vi "TimeTag_LSW_AG_edits_May9.vi"() -> ()   [LabVIEW 2015]
doc: "This sample project is built upon the standard state machine template and shows how you could create an application that acquires, analyzes, and presents data. It includes functionality for presenting configuration dialogs, preserving settings between executions, loading and saving data, as well as exporting graph images and text files.\n\nIt is most appropriate for data that is acquired instantly as it does not allow for screen updates mid acquisition nor does it allow for continuous streaming to disk."
uses:
  <vilib>/ptbypt/NI_PtbyPt.lvlib
panel:
  out "real coin/sec X point average":dbl
  out "Real coin cps X point average":dbl(graph)
  in  "number of points to average real c/s":dbl=100.0
  out "Ch4 100sec avg":dbl
  out "Ch2 100 sec avg":dbl
  out "real coin cps 100 pt\n avg":dbl
  out "all coin cps":dbl
  out "real coin cps":dbl
  out "random coin cps":dbl
  out "Real coin cps":dbl(graph)
  out "total coin/sec - total random coin/sec":dbl
  out "total random coincidences/sec":dbl
  out "Total Coin per sec":dbl
  out "Ch2/4 coin/sec":dbl(graph)
  out "Ch2/4 Total Coincidences":dbl
  out "Channel 2 CPS":dbl(graph)
  out "Channel 4 CPS":dbl(graph)
  out "Total Ch2 CPS":dbl
  out "Total Ch4 CPS":dbl
  in  "Averaging":dbl=10.0
  in  "Runs":dbl=100.0
  in  "Pulse TTL 2":bool
  in  "Pulse TTL 1":bool
  in  "Toggle\nTTL 2":bool
  in  "Toggle\nTTL 1":bool
  out "Total Starts":dbl
  in  "Record data":bool
  out "Initial time":dbl
  out "Elapsed time (s)":dbl
  out "FPGA_Run Status":dbl
  out "USB_Open Status":dbl
  out "Channel 4 Total\nCounts":dbl
  out "Channel 3 Total\nCounts":dbl
  out "Channel 2 Total\nCounts":dbl
  out "Channel 1 Total\nCounts":dbl
  in  "File Name":string="C:\\FPGA\\test.txt"
  out "?":dbl
  out "?":dbl
  out "?":dbl
  out "?":dbl
  out "stats":i64[](array[numeric])
  in  "Stop":bool
  out "Channel 4 CPS":dbl(knob) scale=0.0..2000000.0
  out "Channel 3 CPS":dbl(knob) scale=0.0..600.0
  out "Channel 2 CPS":dbl(knob) scale=0.0..700.0
  out "Channel 1 CPS":dbl(knob) scale=0.0..600.0
  # "Starts"
  # "Channel 1"
  # "Channel 2"
  # "Channel 3"
  # "Channel 4"
  # "Coincidence Channels 1 & 2"
  # "Coincidence Channels 1 & 3"
  # "Coincidence Channels 1 & 4"
  # "Coincidence Channels 2 & 3"
  # "Coincidence Channels 2 & 4"
  # "Coincidence Channels 3 & 4"
  # "Coincidence Channels 1 & 2 & 3"
  # "Coincidence Channels 1 & 2 & 4"
  # "Coincidence Channels 1 & 3 & 4"
  # "Coincidence Channels 2 & 3 & 4"
  # "C:\\FPGA_Lauren"
  # "Coincidence Channels 1 & 2 & 3 & 4"
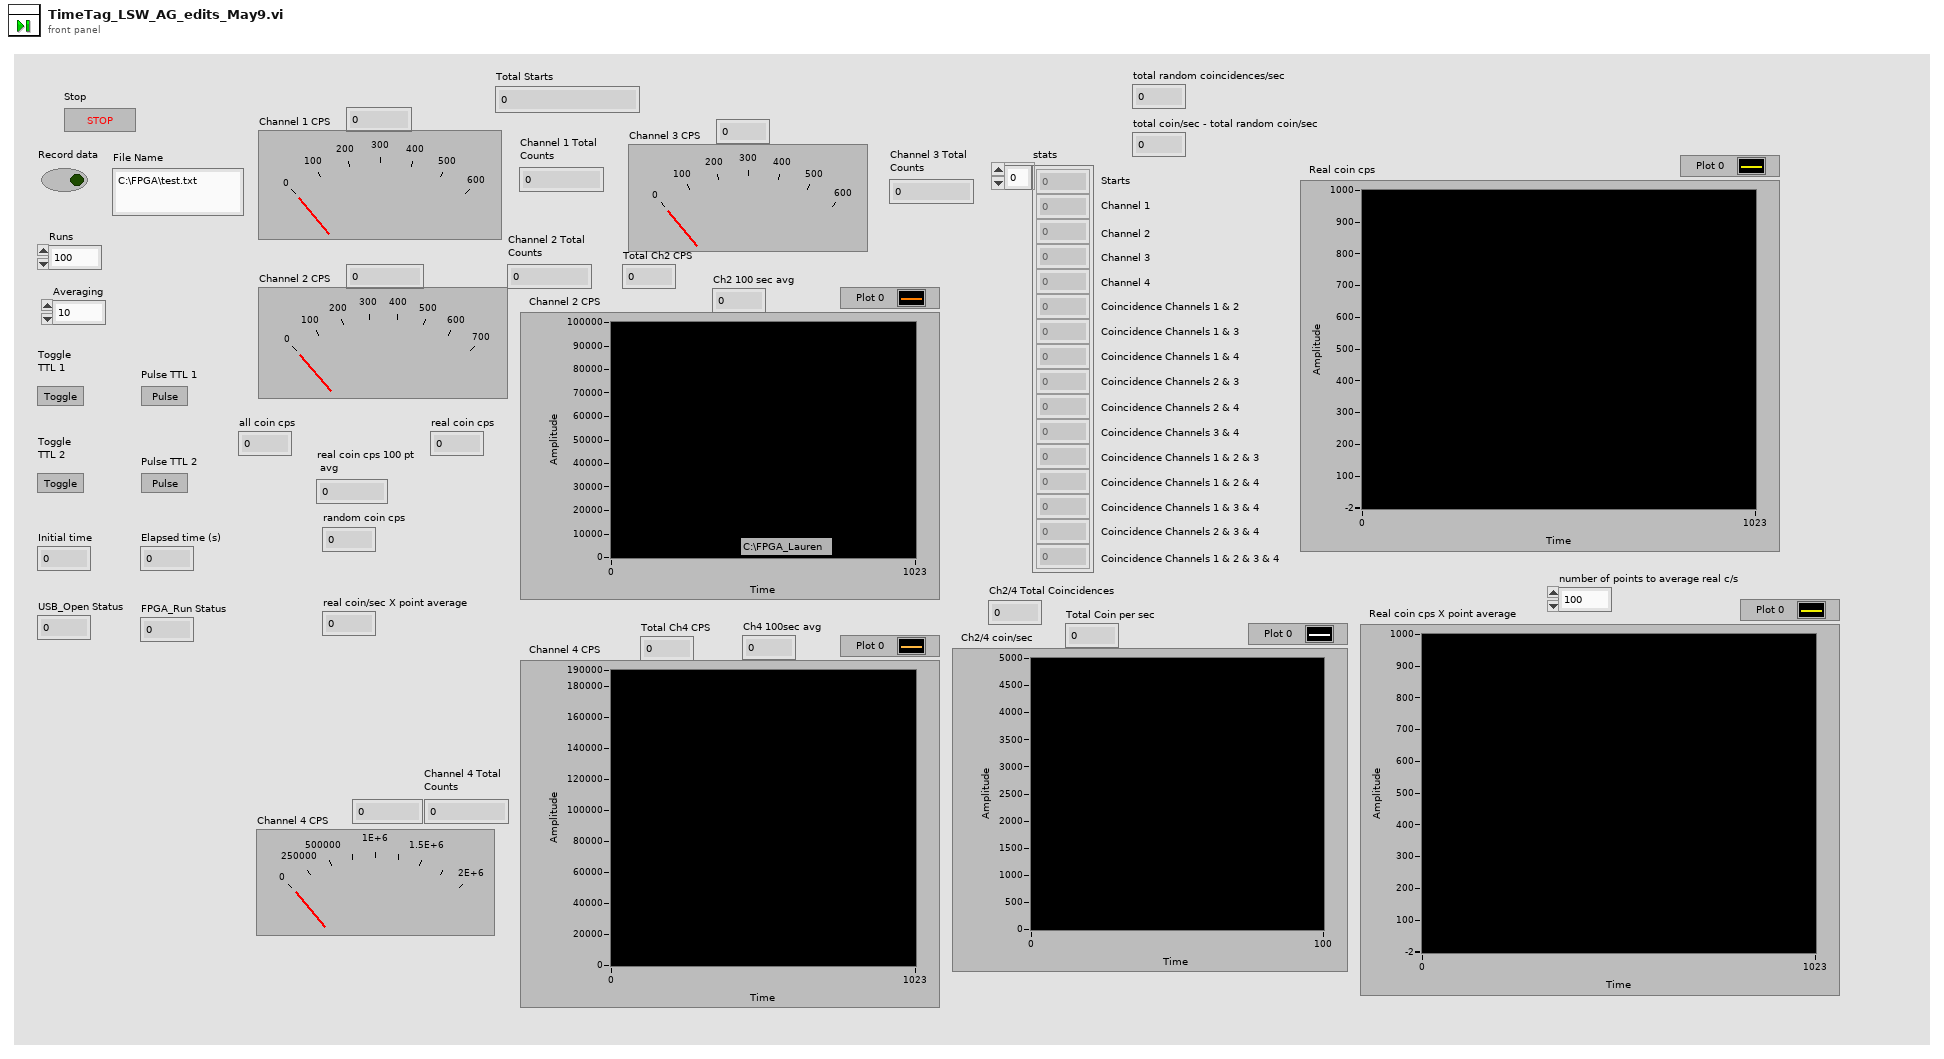
[diagram p1: front panel]
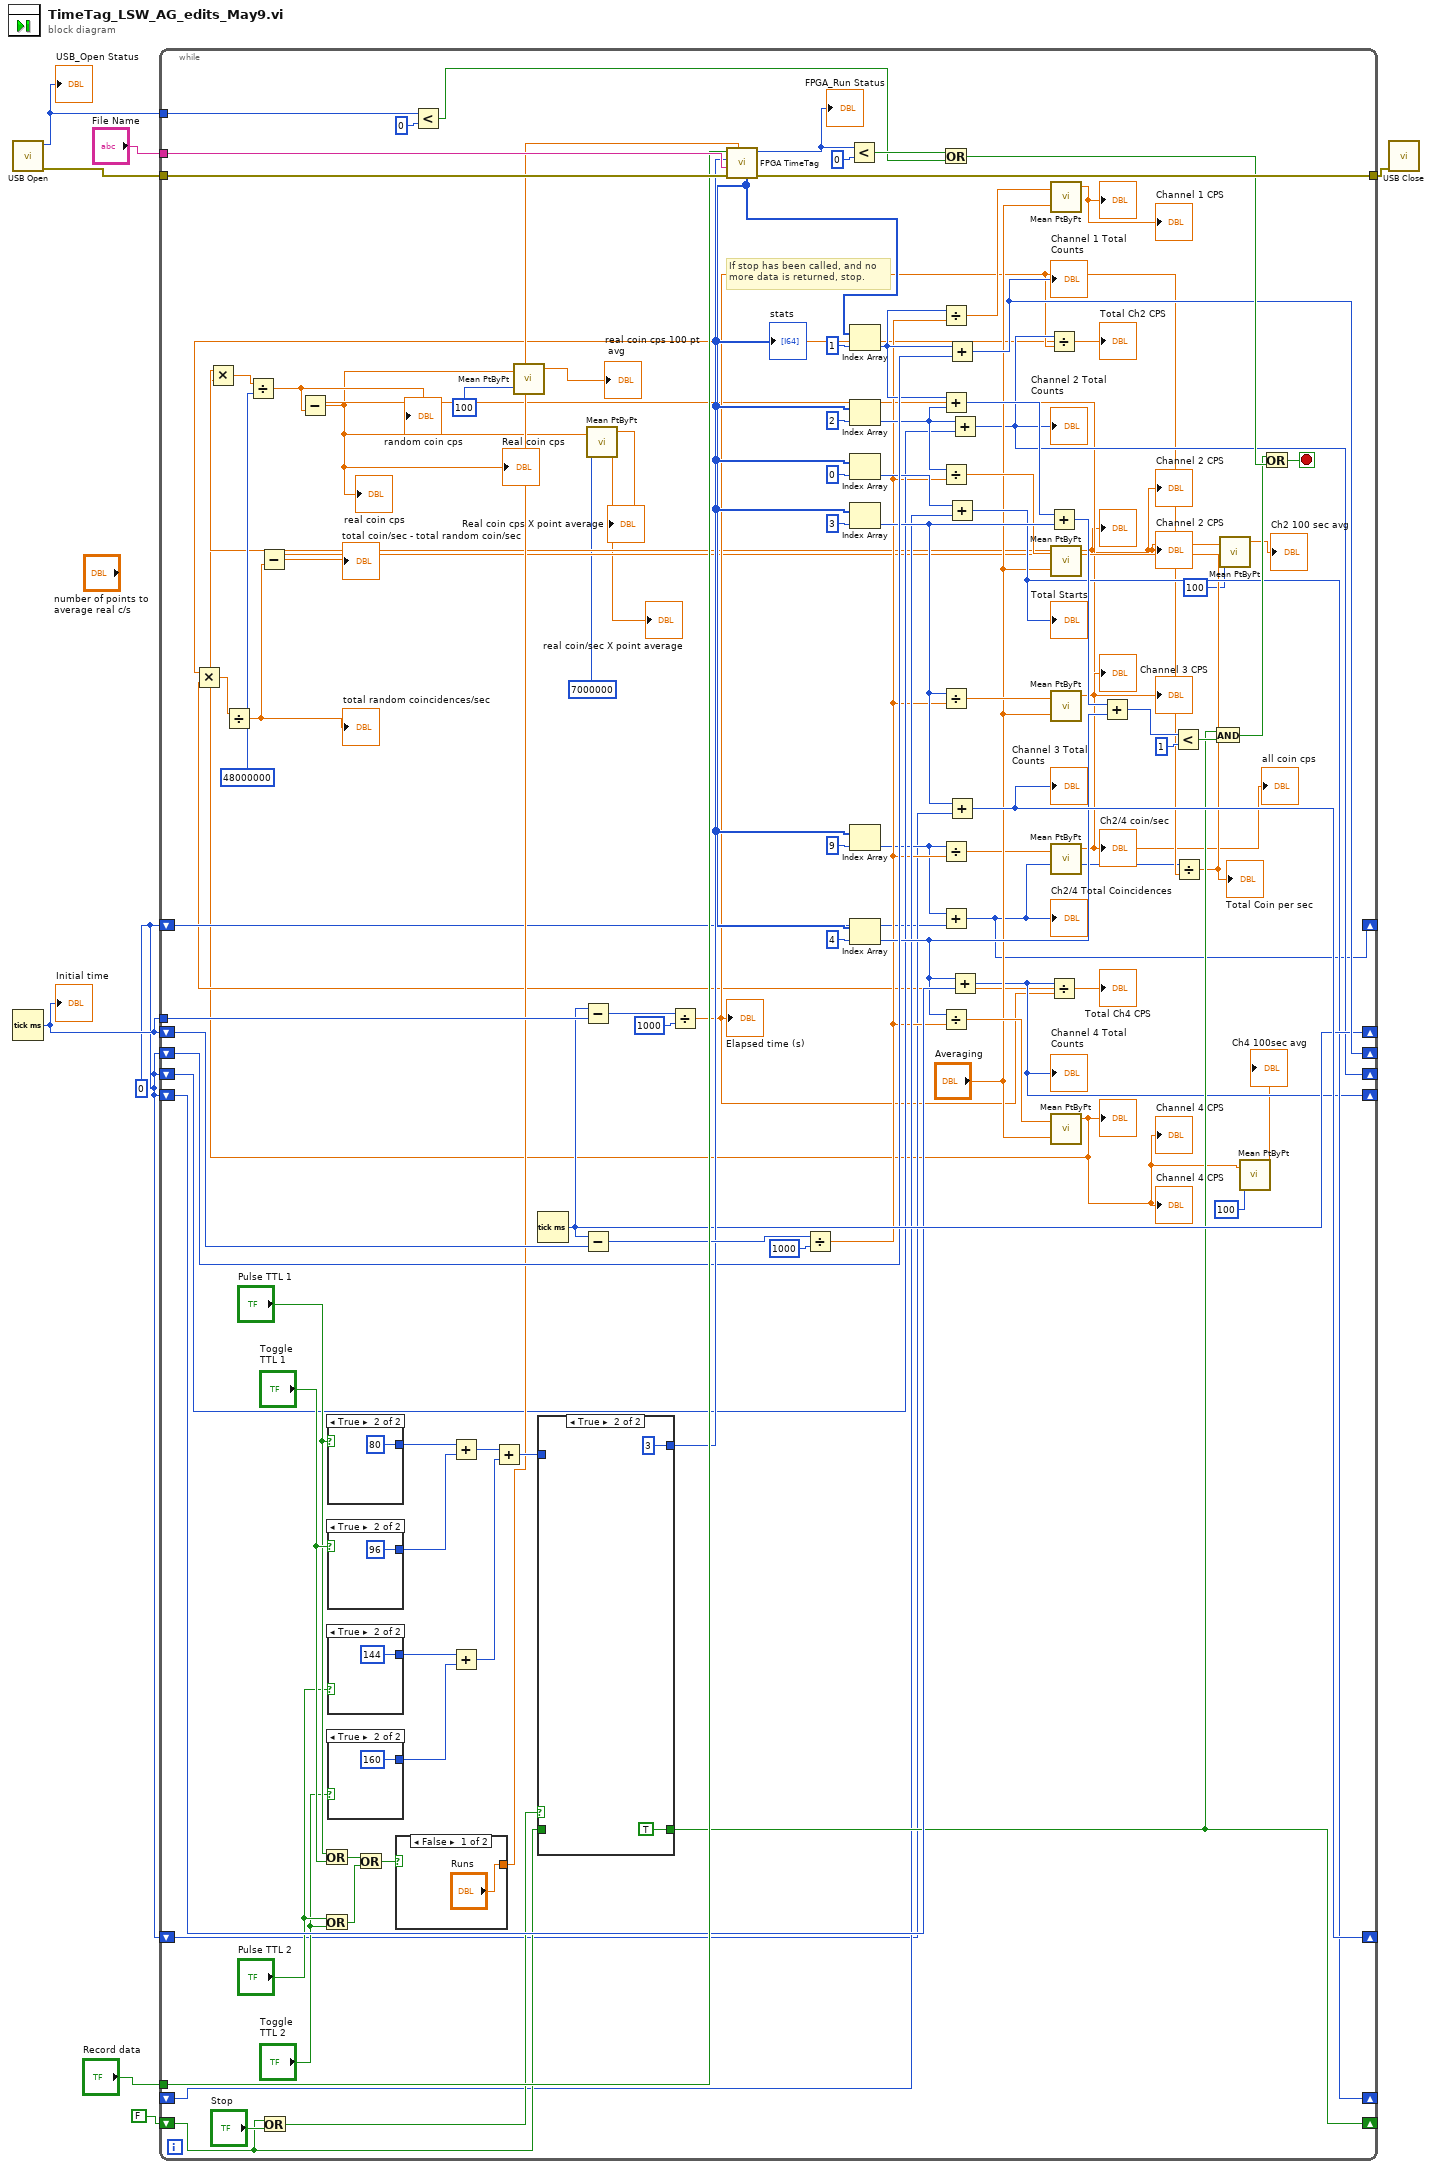
[diagram p0: block diagram]
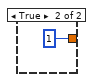
[diagram p2: hidden frame]
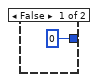
[diagram p3: hidden frame]
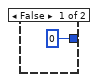
[diagram p4: hidden frame]
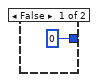
[diagram p5: hidden frame]
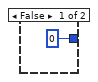
[diagram p6: hidden frame]
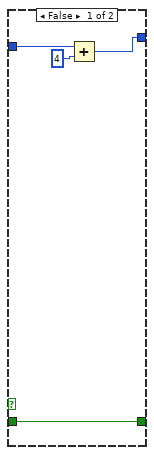
[diagram p7: hidden frame]
diagram:
  w1 = 0
  n1 = call "USB Open.vi"() -> ("error out"=w6:errorcluster, "function return"=w3:i32)  [unwired: 10 in]
  "USB_Open Status" <- w3
  n2 = Tick Count (ms)() -> (millisecond timer value=w4:u32)
  "Initial time" <- w4
  n3 = while {
    tunnel: w4 -> [w109]
    shift-right: [w87] -> _
    shift-left: w1 -> [w83]
    shift-right: [w41] -> _
    shift-left: w1 -> [w37]
    shift-right: [w86] -> _
    shift-left: w1 -> [w33]
    shift-right: [w42] -> _
    shift-left: w1 -> [w82]
    tunnel: w6 -> [w99]
    tunnel: [w100] -> w5
    tunnel: "Record data" -> [w97]
    tunnel: "File Name" -> [w98]
    shift-right: [w84] -> _
    shift-left: w4 -> [w95]
    tunnel: w3 -> [w91]
    shift-right: [w71] -> _
    shift-left: FALSE -> [w68]
    shift-right: [w64] -> _
    shift-left: _ -> [w65]
    shift-right: [w30] -> _
    shift-left: w1 -> [w32]
    stop <- w101 stop-if-true
    w24 = 48000000
    # "If stop has been called, and no\nmore data is returned, stop."
    n4 = Or(x=w68, y="Stop") -> (x .or. y?=w70:bool)
    n5 = Or(x="Pulse TTL 1", y="Toggle\nTTL 1") -> (x .or. y?=w55:bool)
    n6 = Or(x="Pulse TTL 2", y="Toggle\nTTL 2") -> (x .or. y?=w56:bool)
    n7 = case shown="True" "Pulse TTL 1" {
      tunnel: [0 80] -> w63
      frame False {
      }
      frame True {
      }
    }
    n8 = case shown="True" "Toggle\nTTL 1" {
      tunnel: [0 96] -> w62
      frame False {
      }
      frame True {
      }
    }
    n9 = case shown="True" "Pulse TTL 2" {
      tunnel: [0 144] -> w59
      frame False {
      }
      frame True {
      }
    }
    n10 = case shown="True" "Toggle\nTTL 2" {
      tunnel: [0 160] -> w60
      frame False {
      }
      frame True {
      }
    }
    n11 = Or(x=w55, y=w56) -> (x .or. y?=w57:bool)
    n12 = case shown="False" w57 {
      tunnel: ["Runs" 1] -> w53
      frame False {
      }
      frame True {
      }
    }
    n13 = Less?(x=w91, y=0) -> (x < y?=w89:bool)
    n14 = Add(x=w63, y=w62) -> (x+y=w61:i32)
    n15 = Add(x=w59, y=w60) -> (x+y=w58:i32)
    n16 = Add(x=w61, y=w58) -> (x+y=w54:i32)
    n17 = Tick Count (ms)() -> (millisecond timer value=w84:u32)
    n18 = case shown="True" w70 {
      tunnel: [w121 3] -> w85
      tunnel: [w123 TRUE] -> w71
      tunnel: w68 -> [w123 _]
      tunnel: w54 -> [w120 _]
      frame False {
        n19 = Add(x=w120, y=4) -> (x+y=w121:i32)
      }
      frame True {
      }
    }
    n20 = Subtract(x=w84, y=w109) -> (x-y=w108:u32)
    n21 = Subtract(x=w84, y=w95) -> (x-y=w94:u32)
    n22 = Divide(x=w108, y=1000) -> (x/y=w31:dbl)
    "Elapsed time (s)" <- w31
    n23 = call "FPGA TimeTag.vi"("runs"=w53, "error in (no error)"=w99, "fileName"=w98, "fpgaCommand"=w85, "saveData"=w97) -> ("error out"=w100:errorcluster, "function return"=w96:i32, "stats"=w39:i64[])  [unwired: 4 in]
    "stats" <- w39
    "FPGA_Run Status" <- w96
    n24 = Divide(x=w94, y=1000) -> (x/y=w36:dbl)
    n25 = Less?(x=w96, y=0) -> (x < y?=w90:bool)
    n26 = Index Array(array=w39, index=1) -> (element=w74:i64)
    n27 = Index Array(array=w39, index=2) -> (element=w81:i64)
    n28 = Index Array(array=w39, index=0) -> (element=w66:i64)
    n29 = Index Array(array=w39, index=3) -> (element=w77:i64)
    n30 = Index Array(array=w39, index=9) -> (element=w34:i64)
    n31 = Index Array(array=w39, index=4) -> (element=w78:i64)
    n32 = Or(x=w90, y=w89) -> (x .or. y?=w88:bool)
    n33 = Divide(x=w74, y=w36) -> (x/y=w48:dbl)
    n34 = Add(x=w74, y=w81) -> (x+y=w76:i64)
    n35 = Divide(x=w81, y=w36) -> (x/y=w47:dbl)
    n36 = Divide(x=w77, y=w36) -> (x/y=w46:dbl)
    n37 = Divide(x=w34, y=w36) -> (x/y=w35:dbl)
    n38 = Add(x=w34, y=w32) -> (x+y=w30:i64)
    "Ch2/4 Total Coincidences" <- w30
    n39 = Divide(x=w78, y=w36) -> (x/y=w44:dbl)
    n40 = Add(x=w74, y=w83) -> (x+y=w87:i64)
    "Channel 1 Total\nCounts" <- w87
    n41 = Add(x=w66, y=w65) -> (x+y=w64:i64)
    "Total Starts" <- w64
    n42 = Add(x=w77, y=w33) -> (x+y=w86:i64)
    "Channel 3 Total\nCounts" <- w86
    n43 = Add(x=w81, y=w37) -> (x+y=w41:i64)
    "Channel 2 Total\nCounts" <- w41
    n44 = Add(x=w78, y=w82) -> (x+y=w42:i64)
    "Channel 4 Total\nCounts" <- w42
    n45 = Divide(x=w41, y=w31) -> (x/y=w27:dbl)
    "Total Ch2 CPS" <- w27
    n46 = Add(x=w76, y=w77) -> (x+y=w80:i64)
    n47 = Divide(x=w42, y=w31) -> (x/y=w26:dbl)
    "Total Ch4 CPS" <- w26
    n48 = Multiply(x=w27, y=w26) -> (x*y=w25:dbl)
    n49 = Divide(x=w25, y=w24) -> (x/y=w28:dbl)
    "total random coincidences/sec" <- w28
    n50 = call <vilib>:"Mean PtByPt.vi"("x"=w48, "sample length"="Averaging") -> ("mean"=→"Channel 1 CPS" →"?":dbl)  [unwired: 2 in, 1 out]
    n51 = call <vilib>:"Mean PtByPt.vi"("x"=w47, "sample length"="Averaging") -> ("mean"=w17:dbl)  [unwired: 2 in, 1 out]
    "Channel 2 CPS" <- w17
    "?" <- w17
    "Channel 2 CPS" <- w17
    n52 = call <vilib>:"Mean PtByPt.vi"("x"=w46, "sample length"="Averaging") -> ("mean"=→"Channel 3 CPS" →"?":dbl)  [unwired: 2 in, 1 out]
    n53 = call <vilib>:"Mean PtByPt.vi"("x"=w35) -> ("mean"=w20:dbl)  [unwired: 3 in, 1 out]
    "Ch2/4 coin/sec" <- w20
    "all coin cps" <- w20
    n54 = call <vilib>:"Mean PtByPt.vi"("x"=w44, "sample length"="Averaging") -> ("mean"=w14:dbl)  [unwired: 2 in, 1 out]
    "Channel 4 CPS" <- w14
    "?" <- w14
    "Channel 4 CPS" <- w14
    n55 = Multiply(x=w17, y=w14) -> (x*y=w23:dbl)
    n56 = Divide(x=w23, y=w24) -> (x/y=w22:dbl)
    "random coin cps" <- w22
    n57 = Subtract(x=w20, y=w22) -> (x-y=w11:dbl)
    "Real coin cps" <- w11
    "real coin cps" <- w11
    n58 = call <vilib>:"Mean PtByPt.vi"("x"=w11, "sample length"=100) -> ("mean"=→"real coin cps 100 pt\n avg":dbl)  [unwired: 2 in, 1 out]
    n59 = call <vilib>:"Mean PtByPt.vi"("x"=w11, "sample length"=7000000) -> ("mean"=→"Real coin cps X point average" →"real coin/sec X point average":dbl)  [unwired: 2 in, 1 out]
    n60 = Add(x=w80, y=w78) -> (x+y=w79:i64)
    n61 = Less?(x=w79, y=1) -> (x < y?=w73:bool)
    n62 = Divide(x=w30, y=w31) -> (x/y=w29:dbl)
    "Total Coin per sec" <- w29
    n63 = Subtract(x=w29, y=w28) -> (x-y=→"total coin/sec - total random coin/sec":dbl)
    n64 = And(x=w71, y=w73) -> (x .and. y?=w72:bool)
    n65 = call <vilib>:"Mean PtByPt.vi"("x"=w17, "sample length"=100) -> ("mean"=→"Ch2 100 sec avg":dbl)  [unwired: 2 in, 1 out]
    n66 = call <vilib>:"Mean PtByPt.vi"("x"=w14, "sample length"=100) -> ("mean"=→"Ch4 100sec avg":dbl)  [unwired: 2 in, 1 out]
    n67 = Or(x=w72, y=w88) -> (x .or. y?=w101:bool)
  }
  n68 = call "USB Close.vi"("error in (no error)"=w5) -> ()  [unwired: 9 in, 2 out]
